vi "Process triangle.vi"(1 "Triangle in":T1) -> (0 "Triangle out":T1)   [LabVIEW 2014]
doc: "This VI must be run after any alteration to the triangles geometry involving scaling and rotation.\nThere is no need to run this VI after applying a translation."
uses:
  Typedefs/Triangle.ctl
  Subroutines/Dot product.vi
panel:
  # "PN 13/01/2015"
  # "Vertices"
  # "Edges"
  # "Unit normal"
  # "pre-store"
  # "Vertices"
  # "Edges"
  # "Unit normal"
  # "pre-store"
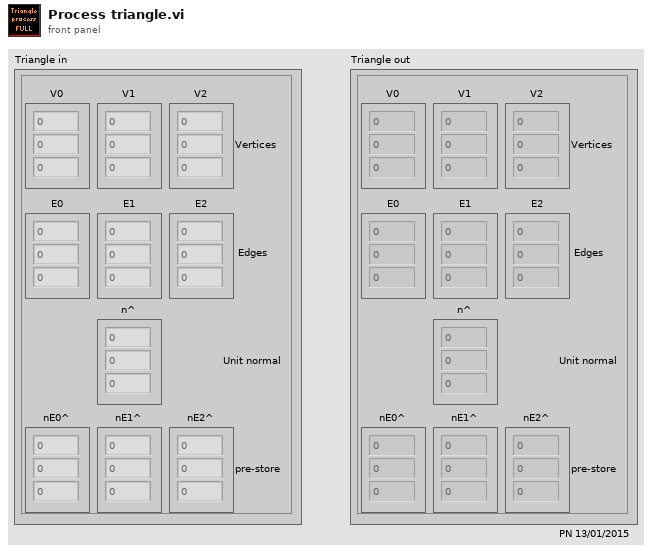
[diagram p1: front panel]
types:
  T1 = typedef "Triangle.ctl" = cluster{"V0":sgl[], "V1":sgl[], "V2":sgl[], "E0":sgl[], "E1":sgl[], "E2":sgl[], "n^":sgl[], "nE0^":sgl[], "nE1^":sgl[], "nE2^":sgl[]}
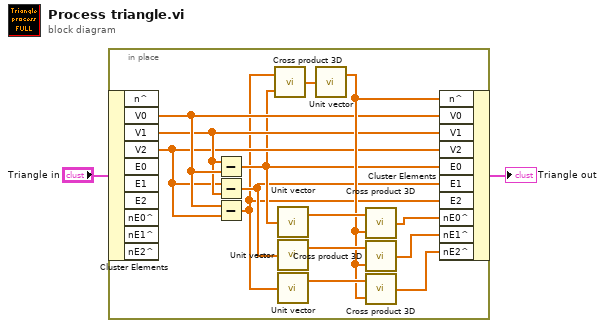
[diagram p0: block diagram]
diagram:
  n1 = in-place {
    n2 = in-place-cluster #1("Triangle in") -> ("V0"=w11:sgl[], "V1"=w10:sgl[], "V2"=w9:sgl[])  [unwired: 7 out]
    n3 = Subtract(x=w10, y=w11) -> (x-y=w8:sgl[])
    n4 = Subtract(x=w9, y=w10) -> (x-y=w7:sgl[])
    n5 = Subtract(x=w11, y=w9) -> (x-y=w6:sgl[])
    n6 = call "Cross product 3D.vi"("B"=w8, "A"=w6) -> ("A x B"=w13:sgl[])
    n7 = call "Unit vector.vi"("Vector"=w8) -> ("Unit vector"=w14:sgl[])  [unwired: 1 out]
    n8 = call "Unit vector.vi"("Vector"=w7) -> ("Unit vector"=w16:sgl[])  [unwired: 1 out]
    n9 = call "Unit vector.vi"("Vector"=w6) -> ("Unit vector"=w15:sgl[])  [unwired: 1 out]
    n10 = call "Unit vector.vi"("Vector"=w13) -> ("Unit vector"=w12:sgl[])  [unwired: 1 out]
    n11 = call "Cross product 3D.vi"("B"=w12, "A"=w14) -> ("A x B"=w5:sgl[])
    n12 = call "Cross product 3D.vi"("B"=w12, "A"=w16) -> ("A x B"=w4:sgl[])
    n13 = call "Cross product 3D.vi"("B"=w12, "A"=w15) -> ("A x B"=w3:sgl[])
    n14 = in-place-cluster #1("n^"=w12, "V0"=w11, "V1"=w10, "V2"=w9, "E0"=w8, "E1"=w7, "E2"=w6, "nE0^"=w5, "nE1^"=w4, "nE2^"=w3) -> (→"Triangle out":T1)
  }
